vi "AddToActionList.vi"(0 "Action":T1 items=["Manual Handshake", "Z Spectroscopy", "DAC Spectroscopy", "Low Frequency Spectroscopy", "External Spectroscopy", "Move Z to Home", "Z Approach"], 5 "error in":T2) -> (14 "Action out":T1 items=["Manual Handshake", "Z Spectroscopy", "DAC Spectroscopy", "Low Frequency Spectroscopy", "External Spectroscopy", "Move Z to Home", "Z Approach"], 19 "error out":T2)   [LabVIEW 2016]
doc: "Adds an action to the list, which is performed at every point in the path list. The possible actions are:\n- 0 -- Handshake\n- 1 -- Z Spectroscopy\n- 2 -- DAC Spectroscopy\n- 3 -- Low Frequency Spectroscopy\n- 4 -- External Spectroscopy\n- 5 -- Move Z to Home\n- 6 -- Z Approach"
uses:
  Controls/Pathmode-Action_Selection.ctl
  Controls/Error_Out.ctl
  Files_ASC500/DLL/ASC500_RemoteControlV27.dll
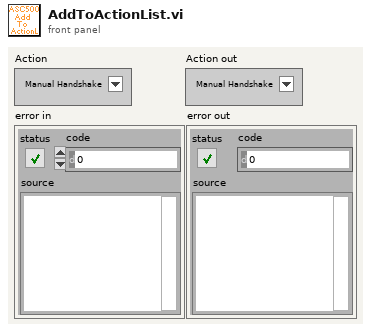
[diagram p1: front panel]
types:
  T1 = typedef "Pathmode-Action_Selection.ctl" = i32
  T2 = typedef "Error_Out.ctl" = errorcluster
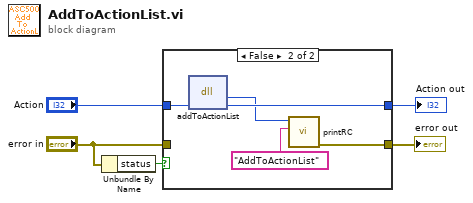
[diagram p0: block diagram]
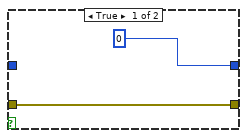
[diagram p2: hidden frame]
diagram:
  n1 = Unbundle By Name("error in") -> ("status"=w5:bool)
  n2 = case shown="False" w5 {
    tunnel: "Action" -> [_ w12]
    tunnel: [0 ("Action") w11] -> w3
    tunnel: [w6 w8] -> w1
    tunnel: "error in" -> [w6 _]
    frame True {
    }
    frame False {
      n3 = dll-call lib="G:/SCMOperations/Share/ELE/Produkt Information/ASC500/04 Remote Control/02 development versions/2018Nov06/Files_ASC500/DLL/ASC500_RemoteControlV27.dll" fn="addToActionList"("Action"=w12) -> ("return type"=w10:i32, "Action"=w11:i32)  [unwired: 3 in, 2 out]
      n4 = call "printRC.vi"("additional information"="AddToActionList", "RC"=w10) -> ("error out"=w8:T2)  [unwired: 9 in]
    }
  }
  "error out" <- w1
  "Action out" <- w3
